vi "Main UI.vi"() -> ()   [LabVIEW 2020]
uses:
  <vilib>/Tag Engine/Tag/Tag.lvclass/Tag.ctl
  02b71a73-c3da-4bb5-9ca2-748e625dec4a.vi
  1fa7eef2-df4a-46ab-87ff-9de60fd7b3df.vi
  8f7cb87c-7f48-47c1-811b-40c30eabf90e.vi
  7d15cc41-90cd-4f37-b1ae-9c20fd0f7ab9.vi
  5d1edfec-8d42-4882-9ca2-830ba54a4b75.vi
  be57360e-2d22-4723-9196-9eb2b215ca80.vi
  14b75dd7-ee25-48f6-8257-ec35bcdfe9bf.vi
  77615359-0bb4-44ca-9655-2864ae5605a2.vi
  7cc18cb2-b148-4661-9fb0-cfe06a915445.vi
  <vilib>/Tag Engine/API/Get Tag Value_ByRef.vi
  <vilib>/Tag Engine/API/Get Tag.vi
  <vilib>/Tag Engine/API/Send Tag SetRequest_ByRef.vi
  <vilib>/Tag Engine/Tag/Read Value.vi
  <vilib>/Tag Engine/Tag/Read Timestamp.vi
  <vilib>/Tag Engine/Tag/Write SetRequest.vi
  <vilib>/Tag Engine/Core/Tag Lookup_By Name.vi
  <vilib>/Tag Engine/Tag Engine.lvlib
  PowerSupply/PowerSupply.lvlib
  <vilib>/Tag Engine/Watchlist/Tag Watchlist.lvlib
  DataLogger/DataLogger.lvlib
  AlarmEngine/AlarmEngine.lvlib
panel:
  in  "Alarms":bool
  out "ALARMS:ALARM1":bool caption="Alarm1"
  out "ALARMS:ALARM2":bool caption="Alarm2"
  in  "LOG1:LOG_EN":bool caption="Logging"
  in  "LOG1:FILE":path
  in  "Stop":bool
  in  "Open Watchlist":bool
  in  "PS1:OUTPUT_EN":bool caption="Output"
  in  "PS1:VOLT_SV":dbl caption="Voltage Amplitude (Peak)" format="%#_g V"
  out "Power Supply 1":cluster{"Value":dbl, "Value":dbl}(graph) caption="Waveform Chart - Dark"
  # "Power Supply 1 Control"
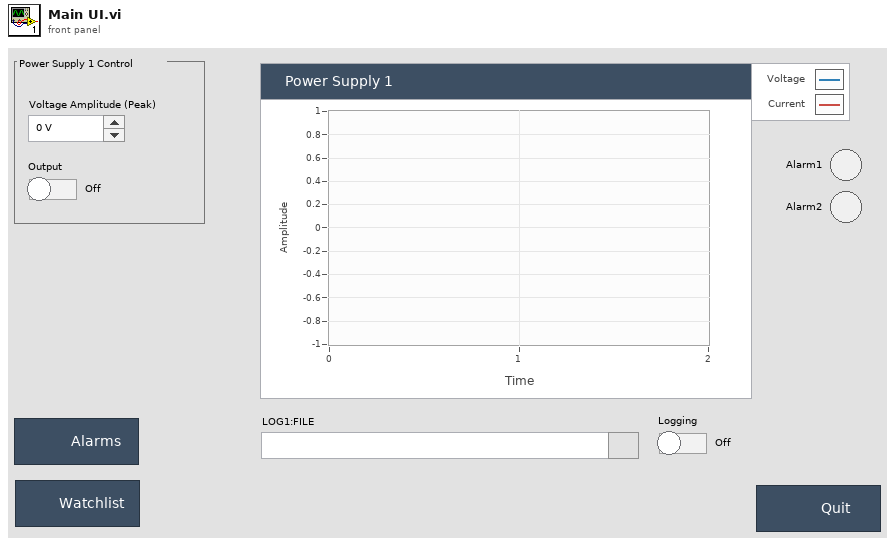
[diagram p1: front panel]
types:
  T1 = cluster{"Alarms":cluster{"Name":string, "Condition":string}[]}
  T2 = cluster{"Vmax":dbl, "Vmin":dbl, "IP Addr":string}
  T3 = cluster{"Default (Void)":dbl, "Default (Void)":dbl}
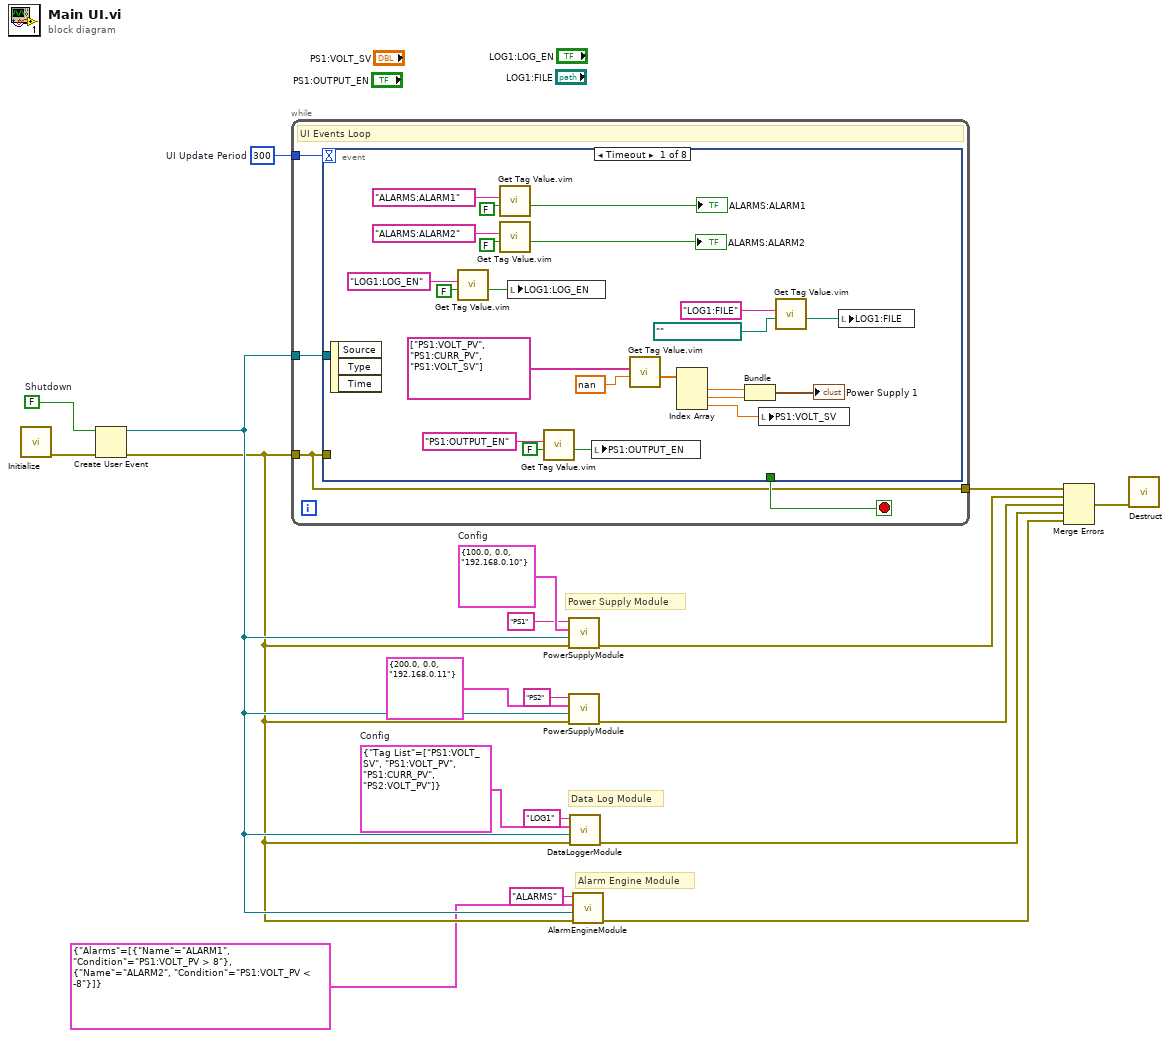
[diagram p0: block diagram]
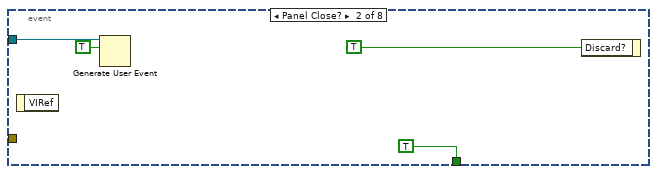
[diagram p2: hidden frame]
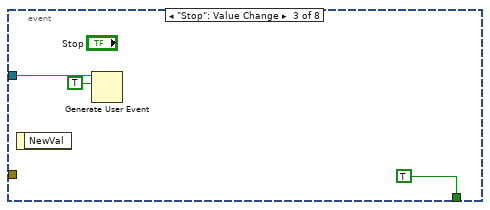
[diagram p3: hidden frame]
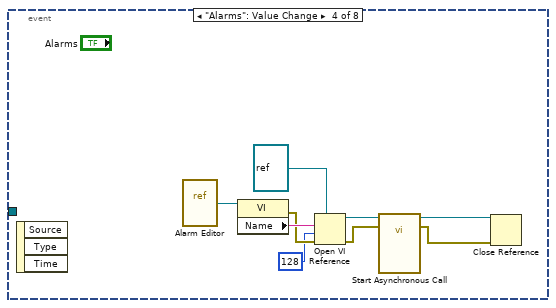
[diagram p4: hidden frame]
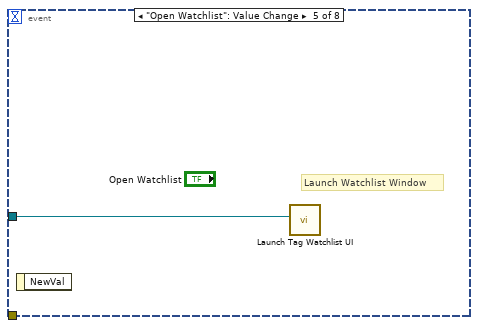
[diagram p5: hidden frame]
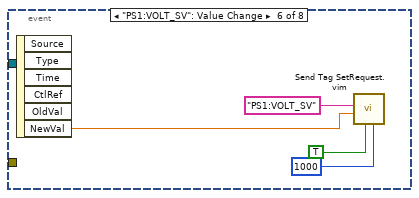
[diagram p6: hidden frame]
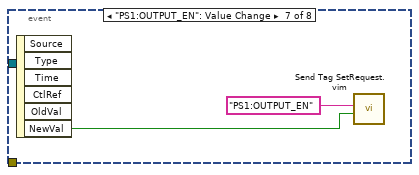
[diagram p7: hidden frame]
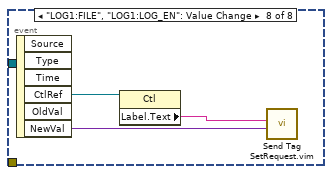
[diagram p8: hidden frame]
diagram:
  w13 = cluster{"Tag List":string[]} {"Tag List"=["PS1:VOLT_SV", "PS1:VOLT_PV", "PS1:CURR_PV", "PS2:VOLT_PV"]}  # Config
  w15 = FALSE  # Shutdown
  w17 = 300  # UI Update Period
  w19 = T2 {"Vmax"=100.0, "Vmin"=0.0, "IP Addr"="192.168.0.10"}  # Config
  # "Alarm Engine Module"
  # "Data Log Module"
  # "Power Supply Module"
  n1 = call <vilib>:"Initialize.vi"() -> ("error out"=w16:errorcluster)  [unwired: 11 in]
  n2 = Create User Event(user event datatype=w15, error in=w16) -> (user event=w7:refnum<user-event>, error out=w6:errorcluster)
  n3 = while {
    tunnel: w17 -> [w22]
    tunnel: w6 -> [w20]
    tunnel: w7 -> [w21]
    tunnel: [w20] -> w12
    stop <- w23 stop-if-true
    # "UI Events Loop"
    n4 = event shown="[0] Timeout" {
      selector: _ -> [_ _ _ _ _ _ _ _]
      dyn-events: _ -> [_ _ _ _ _ _ _ _]
      timeout: w22 -> [_ _ _ _ _ _ _ _]
      tunnel: [_ TRUE TRUE _ _ _ _ _] -> w23
      tunnel: w20 -> [_ _ _ _ _ _ _ _]
      tunnel: w21 -> [_ w46 w51 _ w62 _ _ _]
      event Timeout {
        n5 = event-data() -> ()  [unwired: 1 in, 3 out]
        n6 = call "Get Tag Value.vim"("Default (Void)"=FALSE, "Tag Name(s)/Ref(s)"="LOG1:LOG_EN") -> ("Value(s)"=w35:bool)  [unwired: 6 in, 3 out]
        n7 = call "Get Tag Value.vim"("Default (Void)"=FALSE, "Tag Name(s)/Ref(s)"="ALARMS:ALARM1") -> ("Value(s)"=→"ALARMS:ALARM1":bool)  [unwired: 6 in, 3 out]
        n8 = call "Get Tag Value.vim"("Default (Void)"=FALSE, "Tag Name(s)/Ref(s)"="ALARMS:ALARM2") -> ("Value(s)"=→"ALARMS:ALARM2":bool)  [unwired: 6 in, 3 out]
        n9 = local write "LOG1:LOG_EN"(w35) -> ()
        n10 = call "Get Tag Value.vim"("Default (Void)"=FALSE, "Tag Name(s)/Ref(s)"="PS1:OUTPUT_EN") -> ("Value(s)"=w39:bool)  [unwired: 6 in, 3 out]
        n11 = local write "PS1:OUTPUT_EN"(w39) -> ()
        n12 = call "Get Tag Value.vim"("Default (Void)"=nan, "Tag Name(s)/Ref(s)"=string[] ["PS1:VOLT_PV", "PS1:CURR_PV", "PS1:VOLT_SV"]) -> ("Value(s)"=w30:dbl[])  [unwired: 6 in, 3 out]
        n13 = Index Array(array=w30) -> (element #1=w45:dbl, element #2=w44:dbl, element #3=w42:dbl)  [unwired: 3 in]
        n14 = Bundle("Default (Void)"=w45, "Default (Void)"=w44) -> (→"Power Supply 1":T3)  [unwired: 1 in]
        n15 = local write "PS1:VOLT_SV"(w42) -> ()
        n16 = call "Get Tag Value.vim"("Default (Void)"=path "" ("LOG1:FILE"), "Tag Name(s)/Ref(s)"="LOG1:FILE") -> ("Value(s)"=w37:path)  [unwired: 6 in, 3 out]
        n17 = local write "LOG1:FILE"(w37) -> ()
      }
      event Panel Close? {
        n18 = event-data() -> ()  [unwired: 1 in, 1 out]
        n19 = Generate User Event(user event=w46, event data cluster=TRUE ("event data")) -> ()  [unwired: 2 in, 2 out]
        n20 = event-data("Discard?"=TRUE) -> ()  [unwired: 1 in, 1 out]
      }
      event "Stop": Value Change {
        n21 = event-data() -> ()  [unwired: 1 in, 1 out]
        n22 = Generate User Event(user event=w51, event data cluster=TRUE ("event data")) -> ()  [unwired: 2 in, 2 out]
      }
      event "Alarms": Value Change {
        n23 = event-data() -> ()  [unwired: 1 in, 3 out]
        n24 = vi-ref "Alarm Editor.vi"() -> (w61:refnum<vi>)
        n25 = property class="VI"(reference=w61) -> (error out=w56:errorcluster, "Name"=w60:string)  [unwired: 1 in, 1 out]
        n26 = Open VI Reference(type specifier VI Refnum (for type only)=refnum<vi> refnum, vi path=w60, options=128, error in (no error)=w56) -> (vi reference=w58:refnum<vi>, error out=w54:errorcluster)  [unwired: 2 in]
        n27 = call-by-ref "Start Asynchronous Call"(reference=w58, error in=w54) -> (reference out=w57:refnum<vi>, error out=w53:errorcluster)  [unwired: 12 in]
        n28 = Close Reference(reference=w57, error in (no error)=w53) -> ()  [unwired: 1 out]
      }
      event "Open Watchlist": Value Change {
        # "Launch Watchlist Window"
        n29 = event-data() -> ()  [unwired: 1 in, 1 out]
        n30 = call <vilib>:"Launch Tag Watchlist UI.vi"("Shutdown Event"=w62) -> ()  [unwired: 10 in, 1 out]
      }
      event "PS1:VOLT_SV": Value Change {
        n31 = event-data() -> ("NewVal"=w65:dbl)  [unwired: 1 in, 5 out]
        n32 = call "Send Tag SetRequest.vim"("Timeout (-1)"=1000, "Synchronous (F)"=TRUE, "Value"=w65, "Tag Name(s)/Ref(s)"="PS1:VOLT_SV") -> ()  [unwired: 5 in, 3 out]
      }
      event "PS1:OUTPUT_EN": Value Change {
        n33 = event-data() -> ("NewVal"=w67:bool)  [unwired: 1 in, 5 out]
        n34 = call "Send Tag SetRequest.vim"("Value"=w67, "Tag Name(s)/Ref(s)"="PS1:OUTPUT_EN") -> ()  [unwired: 7 in, 3 out]
      }
      event "LOG1:FILE", "LOG1:LOG_EN": Value Change {
        n35 = event-data() -> ("CtlRef"=w71:refnum<vi>, "NewVal"=w69:variant)  [unwired: 1 in, 4 out]
        n36 = property class="Ctl"(reference=w71) -> ("Label.Text"=w70:string)  [unwired: 1 in, 2 out]
        n37 = call "Send Tag SetRequest.vim"("Value"=w69, "Tag Name(s)/Ref(s)"=w70) -> ()  [unwired: 7 in, 3 out]
      }
    }
  }
  n38 = call "PowerSupplyModule.vi"("error in (no error)"=w6, "Shutdown Event"=w7, "Config"=w19, "ModuleID"="PS1" ("DevID")) -> ("error out"=w11:errorcluster)  [unwired: 7 in]
  n39 = call "PowerSupplyModule.vi"("error in (no error)"=w6, "Shutdown Event"=w7, "Config"=T2 {"Vmax"=200.0, "Vmin"=0.0, "IP Addr"="192.168.0.11"}, "ModuleID"="PS2" ("DevID")) -> ("error out"=w1:errorcluster)  [unwired: 7 in]
  n40 = call "DataLoggerModule.vi"("error in (no error)"=w6, "Shutdown Event"=w7, "Config"=w13, "ModuleID"="LOG1") -> ("error out"=w2:errorcluster)  [unwired: 7 in]
  n41 = call "AlarmEngineModule.vi"("error in (no error)"=w6, "Shutdown Event"=w7, "Config"=T1 {"Alarms"=[{"Name"="ALARM1", "Condition"="PS1:VOLT_PV > 8"}, {"Name"="ALARM2", "Condition"="PS1:VOLT_PV < -8"}]}, "ModuleID"="ALARMS") -> ("error out"=w3:errorcluster)  [unwired: 7 in]
  n42 = Merge Errors(w12, w11, w1, w2, w3) -> (w10:errorcluster)
  n43 = call <vilib>:"Destruct.vi"("error in (no error)"=w10) -> ()  [unwired: 10 in, 1 out]
